vi "Write NumberOfTactics.vi"(8 "error in (no error)":errorcluster, 10 "NumberOfTactics":dbl=3.0, 11 "ABCSecondKicker in":refnum<class "ABCSecondKicker.lvclass">) -> (0 "error out":errorcluster, 3 "ABCSecondKicker out":refnum<class "ABCSecondKicker.lvclass">)   [LabVIEW 2020, in "ABCSecondKicker.lvclass"]
uses:
  ABCSecondKicker.lvclass
  ABCSecondKicker.lvclass/ABCSecondKicker.ctl
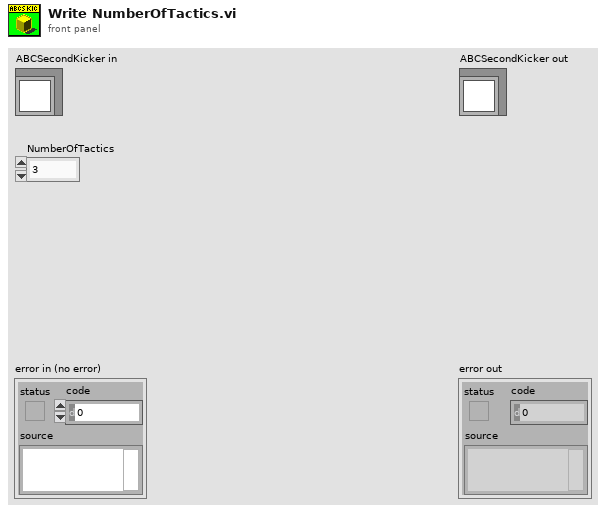
[diagram p1: front panel]
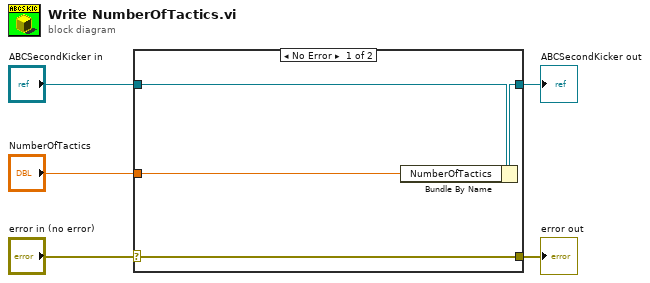
[diagram p0: block diagram]
diagram:
  n1 = case shown="No Error" "error in (no error)" {
    selector: "error in (no error)" -> [w9 w10]
    tunnel: [w9 w10] -> w4
    tunnel: [w7 w11] -> w2
    tunnel: "ABCSecondKicker in" -> [w8 w11]
    tunnel: "NumberOfTactics" -> [w6 _]
    frame No Error {
      n2 = Bundle By Name(cluster=w8, "NumberOfTactics"=w6) -> (w7:refnum<class "ABCSecondKicker.lvclass">)
    }
    frame Error {
    }
  }
  "error out" <- w4
  "ABCSecondKicker out" <- w2
